vi "Maxi Gauge-convert6Flt.vi"(1 "String in":string) -> (4 "Fract1 out":dbl format="%.3f", 6 "Fract2 out":dbl format="%.3f", 8 "Fract3 out":dbl format="%.3f", 10 "Fract4 out":dbl format="%.3f", 14 "Fract6 out":dbl format="%.3f", 15 "Fract5 out":dbl format="%.3f")   [LabVIEW 2012, in "Maxi Gauge.lvlib"]
uses:
  Maxi Gauge.lvlib
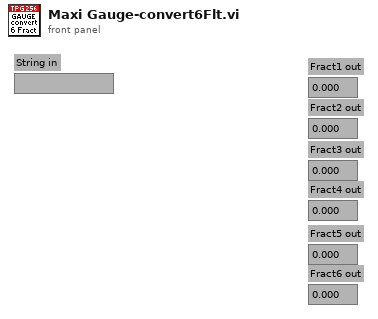
[diagram p1: front panel]
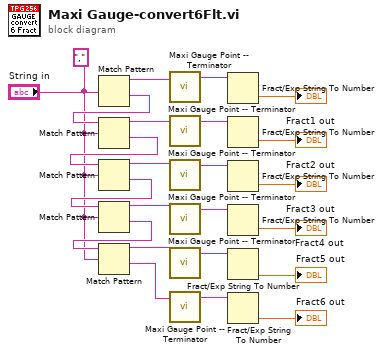
[diagram p0: block diagram]
diagram:
  w1 = "," ("regular expression")
  n1 = Match Pattern(string="String in", regular expression=w1) -> (before substring=w6:string, after substring=w2:string)  [unwired: 1 in, 2 out]
  n2 = Match Pattern(string=w2, regular expression=w1) -> (before substring=w7:string, after substring=w3:string)  [unwired: 1 in, 2 out]
  n3 = Match Pattern(string=w3, regular expression=w1) -> (before substring=w8:string, after substring=w4:string)  [unwired: 1 in, 2 out]
  n4 = Match Pattern(string=w4, regular expression=w1) -> (before substring=w9:string, after substring=w5:string)  [unwired: 1 in, 2 out]
  n5 = Match Pattern(string=w5, regular expression=w1) -> (before substring=w10:string, after substring=w11:string)  [unwired: 1 in, 2 out]
  n6 = call "Maxi Gauge Point -- Terminator.vi"("Eingangstring"=w6) -> ("Ausgangstring"=w12:string)
  n7 = call "Maxi Gauge Point -- Terminator.vi"("Eingangstring"=w7) -> ("Ausgangstring"=w13:string)
  n8 = call "Maxi Gauge Point -- Terminator.vi"("Eingangstring"=w8) -> ("Ausgangstring"=w14:string)
  n9 = call "Maxi Gauge Point -- Terminator.vi"("Eingangstring"=w9) -> ("Ausgangstring"=w15:string)
  n10 = call "Maxi Gauge Point -- Terminator.vi"("Eingangstring"=w10) -> ("Ausgangstring"=w16:string)
  n11 = call "Maxi Gauge Point -- Terminator.vi"("Eingangstring"=w11) -> ("Ausgangstring"=w17:string)
  n12 = Fract/Exp String To Number(string=w12) -> (number=→"Fract1 out":dbl)  [unwired: 3 in, 1 out]
  n13 = Fract/Exp String To Number(string=w13) -> (number=→"Fract2 out":dbl)  [unwired: 3 in, 1 out]
  n14 = Fract/Exp String To Number(string=w14) -> (number=→"Fract3 out":dbl)  [unwired: 3 in, 1 out]
  n15 = Fract/Exp String To Number(string=w15) -> (number=→"Fract4 out":dbl)  [unwired: 3 in, 1 out]
  n16 = Fract/Exp String To Number(string=w16) -> (number=→"Fract5 out":dbl)  [unwired: 3 in, 1 out]
  n17 = Fract/Exp String To Number(string=w17) -> (number=→"Fract6 out":dbl)  [unwired: 3 in, 1 out]
